vi "GOOP_AllVIs.vi"   [LabVIEW 2020]
uses:
  <resource>/Framework/Providers/Open_GDS/SubVIs/GOOP_HelpButton.ctl
  <resource>/Framework/Providers/Open_GDS/SubVIs/GOOP_MethodArgumentConnectionType.ctl
  <resource>/Framework/Providers/Open_GDS/ClassProviders/Common/CommonVIs/CommonVIs_AttributeDataType.ctl
  <resource>/Framework/Providers/Open_GDS/SubVIs/GOOP_MethodArgumentType.ctl
  <resource>/Framework/Providers/Open_GDS/SubVIs/GOOP_ProductType.ctl
  <resource>/Framework/Providers/Open_GDS/SubVIs/GOOP_ToolVersion.vi
  <resource>/Framework/Providers/Open_GDS/SubVIs/GOOP_UMLEditor_CallMainAction.ctl
  <resource>/Framework/Providers/Open_GDS/SubVIs/GOOP_WirePattern.ctl
  <resource>/Framework/Providers/Open_GDS/SubVIs/GOOP_WireConfigurationType.ctl
  <resource>/Framework/Providers/Open_GDS/ClassProviders/Provider_EndevoGOOP300/ClassWriterGOOP300_class/ClassWriterGOOP300.lvclass
  <resource>/Framework/Providers/Open_GDS/SubVIs/GOOP_ClassProviderClassType.ctl
  <resource>/Framework/Providers/Open_GDS/SubVIs/GOOP_ClassSettingsMemory_Action.ctl
  <resource>/Framework/Providers/Open_GDS/ClassProviders/Provider_LvNativeClass/ClassWriterNative_class/ClassWriterNative.lvclass
  <resource>/Framework/Providers/Open_GDS/SubVIs/GOOP_ErrorCodes.ctl
types:
  T1 = typedef "GOOP_ErrorCodes.ctl" = enum16{"LicenseFileMissing", "LicenseFileNotCorrect", "NoProductAccessGranted", "AgreementNoAccepted", "NoValidProviderFound", "LicenseExpired", "LanguageUndefined", "LanguageFileMissing", "LanguageFileChecksumError", "DublicateLanguageTranslation", "LanguageStringIDNotFound", "CommunityLimitReached", "ClassFileLocked", "ClassFileReadOnly", "ProjectNotValid"}
  T2 = typedef "GOOP_ClassSettingsMemory_Action.ctl" = enum16{"Read", "Write", "Read (ClassItemIconOnly)"}
  T3 = typedef "GOOP_ClassProviderClassType.ctl" = enum16{"ClassWriter", "ClassReader"}
  T4 = typedef "GOOP_WirePattern.ctl" = enum16{"Solid", "Large dash", "Small dash"}
  T5 = typedef "GOOP_WireConfigurationType.ctl" = cluster{"Edge thickness":i32, "Edge color":u32, "Center thickness":i32, "Center pattern":T4, "CenterColor1":u32, "CenterColor2":u32, "Tunnels and terminals colors":u32}
  T6 = typedef "GOOP_UMLEditor_CallMainAction.ctl" = enum16{"OpenUmlEditor", "ReverseEngineering:WholeProject", "ReverseEngineering:OneClass", "ReverseEngineering:OneVI", "ShowInStateDiagram:OneVI", "OpenUMLFile"}
  T7 = typedef "GOOP_ProductType.ctl" = enum16{"InvalidType", "Community Edition", "Professional Edition", "UML Community Edition", "UML Architect Edition"}
  T8 = typedef "GOOP_MethodArgumentType.ctl" = cluster{"Name":string, "DataType":T9, "ArrayDimensions":u8, "ConnectionType":T10, "DataTypeReference":path}
  T9 = typedef "CommonVIs_AttributeDataType.ctl" = enum16{"UINT8", "INT8", "UINT16", "INT16", "UINT32", "INT32", "UINT64", "INT64", "SGL", "DBL", "EXT", "CSG", "CDB", "CXT", "TimeStamp", "STRING", "PATH", "BOOL", "ENUM", "RefNum", "VIRefNum", "LabVIEW Class", "Cluster", "Variant", "TypeDef", "Waveform", "LabVIEW Object", "Other", "void", "Set", "Map"}
  T10 = typedef "GOOP_MethodArgumentConnectionType.ctl" = enum16{"Required", "Recommended", "Optional", "Dynamic Dispatch"}
  T11 = typedef "GOOP_HelpButton.ctl" = bool
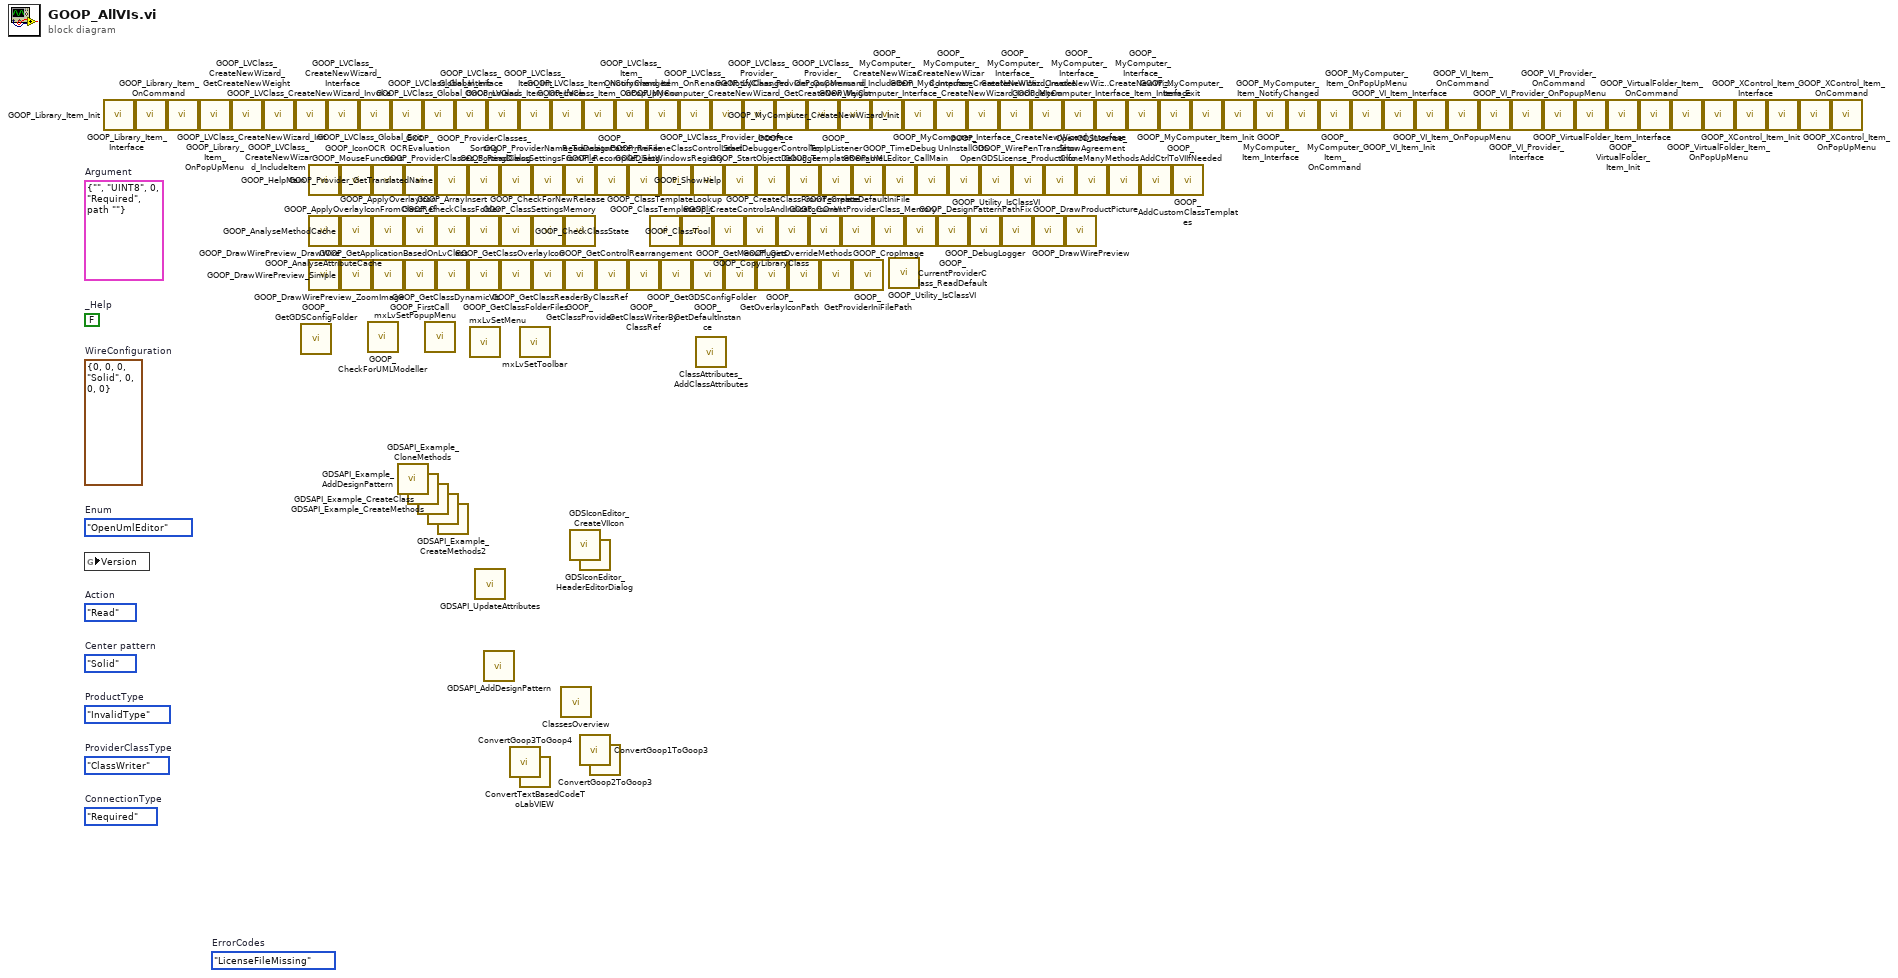
[diagram p0: block diagram]
diagram:
  (unwired) GOOP_ErrorCodes."LicenseFileMissing"  # ErrorCodes
  (unwired) GOOP_ClassSettingsMemory_Action."Read"  # Action
  (unwired) GOOP_ClassProviderClassType."ClassWriter"  # ProviderClassType
  (unwired) GOOP_WirePattern."Solid"  # Center pattern
  (unwired) T5 {"Edge thickness"=0, "Edge color"=0, "Center thickness"=0, "Center pattern"=enum."Solid", "CenterColor1"=0, "CenterColor2"=0, "Tunnels and terminals colors"=0}  # WireConfiguration
  (unwired) GOOP_UMLEditor_CallMainAction."OpenUmlEditor"  # Enum
  (unwired) GOOP_ProductType."InvalidType"  # ProductType
  (unwired) T8 {"Name"="", "DataType"=enum."UINT8", "ArrayDimensions"=0, "ConnectionType"=enum."Required", "DataTypeReference"=path ""}  # Argument
  (unwired) GOOP_MethodArgumentConnectionType."Required"  # ConnectionType
  (unwired) T11 FALSE  # _Help
  n1 = global read "GOOP_ToolVersion.vi" "Version"() -> ()  [unwired: 1 in]
  n2 = call <resource>:"GOOP_Library_Item_Init.vi"() -> ()  [unwired: 12 in]
  n3 = call <resource>:"GOOP_Library_Item_Interface.vi"() -> ()  [unwired: 11 in, 1 out]
  n4 = call <resource>:"GOOP_Library_Item_OnCommand.vi"() -> ()  [unwired: 12 in]
  n5 = call <resource>:"GOOP_Library_Item_OnPopUpMenu.vi"() -> ()  [unwired: 12 in]
  n6 = call <resource>:"GOOP_LVClass_CreateNewWizard_GetCreateNewWeight.vi"() -> ()  [unwired: 11 in, 1 out]
  n7 = call <resource>:"GOOP_LVClass_CreateNewWizard_IncludeItem.vi"() -> ()  [unwired: 11 in, 1 out]
  n8 = call <resource>:"GOOP_LVClass_CreateNewWizard_Init.vi"() -> ()  [unwired: 9 in, 3 out]
  n9 = call <resource>:"GOOP_GetGDSConfigFolder.vi"() -> ()  [unwired: 1 out]
  n10 = call <resource>:"GOOP_HelpMain.vi"() -> ()  [unwired: 12 in]
  n11 = call <resource>:"GOOP_AnalyseAttributeCache.vi"() -> ()  [unwired: 9 in, 3 out]
  n12 = call <resource>:"GOOP_DrawWirePreview_DrawWire.vi"() -> ()  [unwired: 11 in, 1 out]
  n13 = call <resource>:"GOOP_LVClass_CreateNewWizard_Interface.vi"() -> ()  [unwired: 11 in, 1 out]
  n14 = call <resource>:"GOOP_IconOCR.vi"() -> ()  [unwired: 11 in, 1 out]
  n15 = call <resource>:"GOOP_AnalyseMethodCache.vi"() -> ()  [unwired: 9 in, 3 out]
  n16 = call <resource>:"GOOP_DrawWirePreview_Simple.vi"() -> ()  [unwired: 7 in, 5 out]
  n17 = call <resource>:"GOOP_LVClass_CreateNewWizard_Invoke.vi"() -> ()  [unwired: 11 in, 1 out]
  n18 = call <resource>:"GOOP_CheckForUMLModeller.vi"() -> ()  [unwired: 10 in, 2 out]
  n19 = call <resource>:"GOOP_MouseFunctions.vi"() -> ()  [unwired: 9 in, 3 out]
  n20 = call <resource>:"GOOP_ApplyOverlayIcon.vi"() -> ()  [unwired: 11 in, 1 out]
  n21 = call <resource>:"GOOP_DrawWirePreview_ZoomImage.vi"() -> ()  [unwired: 2 in, 1 out]
  n22 = call <resource>:"GOOP_LVClass_Global_Exit.vi"() -> ()  [unwired: 12 in]
  n23 = call <resource>:"GDSAPI_Example_AddDesignPattern.vi"() -> ()  [unwired: 12 in]
  n24 = call <resource>:"GOOP_OCREvaluation.vi"() -> ()  [unwired: 11 in, 1 out]
  n25 = call <resource>:"GOOP_ApplyOverlayIconFromClassRef.vi"() -> ()  [unwired: 11 in, 1 out]
  n26 = call <resource>:"GOOP_FirstCall.vi"() -> ()  [unwired: 11 in, 1 out]
  n27 = call <resource>:"GDSAPI_Example_CloneMethods.vi"() -> ()  [unwired: 12 in]
  n28 = call <resource>:"GDSAPI_Example_CreateClass.vi"() -> ()  [unwired: 12 in]
  n29 = call <resource>:"GOOP_LVClass_Global_Init.vi"() -> ()  [unwired: 12 in]
  n30 = call <resource>:"mxLvSetPopupMenu.vi"() -> ()  [unwired: 10 in, 2 out]
  n31 = call <resource>:"GDSAPI_Example_CreateMethods.vi"() -> ()  [unwired: 12 in]
  n32 = call <resource>:"GOOP_Provider_GetTranslatedName.vi"() -> ()  [unwired: 11 in, 1 out]
  n33 = call <resource>:"GOOP_ArrayInsert.vi"() -> ()  [unwired: 19 in, 1 out]
  n34 = call <resource>:"GOOP_GetApplicationBasedOnLvClass.vi"() -> ()  [unwired: 10 in, 2 out]
  n35 = call <resource>:"GDSAPI_Example_CreateMethods2.vi"() -> ()  [unwired: 12 in]
  n36 = call <resource>:"GOOP_LVClass_Global_Interface.vi"() -> ()  [unwired: 11 in, 1 out]
  n37 = call <resource>:"GOOP_ProviderClasses_Sorting.vi"() -> ()  [unwired: 9 in, 3 out]
  n38 = call <resource>:"GOOP_CheckClassFolder.vi"() -> ()  [unwired: 7 in, 5 out]
  n39 = call <resource>:"GOOP_GetClassDynamicVIs.vi"() -> ()  [unwired: 12 in, 8 out]
  n40 = call <resource>:"mxLvSetMenu.vi"() -> ()  [unwired: 10 in, 2 out]
  n41 = call <resource>:"GDSAPI_UpdateAttributes.vi"() -> ()  [unwired: 11 in, 1 out]
  n42 = call <resource>:"GDSAPI_AddDesignPattern.vi"() -> ()  [unwired: 11 in, 1 out]
  n43 = call <resource>:"GOOP_LVClass_Global_OnCommand.vi"() -> ()  [unwired: 12 in]
  n44 = call <resource>:"GOOP_ProviderClasses_SortingDialog.vi"() -> ()  [unwired: 9 in, 3 out]
  n45 = call <resource>:"GOOP_CheckClassState.vi"() -> ()  [unwired: 11 in, 1 out]
  n46 = call <resource>:"GOOP_GetClassFolderFiles.vi"() -> ()  [unwired: 11 in, 1 out]
  n47 = call <resource>:"ConvertGoop3ToGoop4.vi"() -> ()  [unwired: 11 in, 1 out]
  n48 = call <resource>:"GOOP_LVClass_Item_Init.vi"() -> ()  [unwired: 12 in]
  n49 = call <resource>:"mxLvSetToolbar.vi"() -> ()  [unwired: 10 in, 2 out]
  n50 = call <resource>:"ConvertTextBasedCodeToLabVIEW.vi"() -> ()  [unwired: 12 in]
  n51 = call <resource>:"GOOP_ProviderName_Translator.vi"() -> ()  [unwired: 11 in, 1 out]
  n52 = call <resource>:"GOOP_CheckForNewRelease.vi"() -> ()  [unwired: 12 in]
  n53 = call <resource>:"GOOP_GetClassOverlayIcon.vi"() -> ()  [unwired: 9 in, 3 out]
  n54 = call <resource>:"GOOP_LVClass_Item_Interface.vi"() -> ()  [unwired: 11 in, 1 out]
  n55 = call <resource>:"ClassesOverview.vi"() -> ()  [unwired: 11 in, 1 out]
  n56 = call <resource>:"GOOP_ReadClassSettingsFromFile.vi"() -> ()  [unwired: 9 in, 3 out]
  n57 = call <resource>:"GOOP_ClassSettingsMemory.vi"() -> ()  [unwired: 14 in, 6 out]
  n58 = call <resource>:"GOOP_GetClassProvider.vi"() -> ()  [unwired: 17 in, 3 out]
  n59 = call <resource>:"GDSIconEditor_CreateVIIcon.vi"() -> ()  [unwired: 11 in, 1 out]
  n60 = call <resource>:"GDSIconEditor_HeaderEditorDialog.vi"() -> ()  [unwired: 15 in, 5 out]
  n61 = call <resource>:"ConvertGoop1ToGoop3.vi"() -> ()  [unwired: 11 in, 1 out]
  n62 = call <resource>:"GOOP_LVClass_Item_NotifyChanged.vi"() -> ()  [unwired: 12 in]
  n63 = call <resource>:"ConvertGoop2ToGoop3.vi"() -> ()  [unwired: 11 in, 1 out]
  n64 = call <resource>:"GOOP_ReadDesignPatternIniFile.vi"() -> ()  [unwired: 10 in, 2 out]
  n65 = call <resource>:"GOOP_GetClassReaderByClassRef.vi"() -> ()  [unwired: 18 in, 2 out]
  n66 = call <resource>:"GOOP_LVClass_Item_OnCommand.vi"() -> ()  [unwired: 12 in]
  n67 = call <resource>:"GOOP_RecompileDialog.vi"() -> ()  [unwired: 19 in, 1 out]
  n68 = call <resource>:"GOOP_GetClassWriterByClassRef.vi"() -> ()  [unwired: 18 in, 2 out]
  n69 = call <resource>:"GOOP_LVClass_Item_OnPopUpMenu.vi"() -> ()  [unwired: 12 in]
  n70 = call <resource>:"GOOP_ClassTemplateLookup.vi"() -> ()  [unwired: 11 in, 1 out]
  n71 = call <resource>:"GOOP_RenameClassControlLabel.vi"() -> ()  [unwired: 10 in, 2 out]
  n72 = call <resource>:"GOOP_GetControlRearrangement.vi"() -> ()  [unwired: 13 in, 7 out]
  n73 = call <resource>:"GOOP_LVClass_Item_OnRename.vi"() -> ()  [unwired: 12 in]
  n74 = call <resource>:"GOOP_ClassTemplateSplit.vi"() -> ()  [unwired: 14 in, 2 out]
  n75 = call <resource>:"GOOP_SetWindowsRegistry.vi"() -> ()  [unwired: 11 in, 1 out]
  n76 = call <resource>:"GOOP_GetDefaultInstance.vi"() -> ()  [unwired: 9 in, 3 out]
  n77 = call <resource>:"ClassAttributes_AddClassAttributes.vi"() -> ()  [unwired: 8 in, 4 out]
  n78 = call <resource>:"GOOP_LVClass_Provider_Interface.vi"() -> ()  [unwired: 11 in, 1 out]
  n79 = call <resource>:"GOOP_ClassTool.vi"() -> ()  [unwired: 19 in, 1 out]
  n80 = call <resource>:"GOOP_ShowHelp.vi"() -> ()  [unwired: 1 in]
  n81 = call <resource>:"GOOP_GetGDSConfigFolder.vi"() -> ()  [unwired: 1 out]
  n82 = call <resource>:"GOOP_LVClass_Provider_NotifyChanged.vi"() -> ()  [unwired: 12 in]
  n83 = call <resource>:"GOOP_CopyLibraryClass.vi"() -> ()  [unwired: 9 in, 3 out]
  n84 = call <resource>:"GOOP_StartDebuggerController.vi"() -> ()  [unwired: 19 in, 1 out]
  n85 = call <resource>:"GOOP_GetMenuPlugins.vi"() -> ()  [unwired: 10 in, 2 out]
  n86 = call <resource>:"GOOP_LVClass_Provider_OnCommand.vi"() -> ()  [unwired: 12 in]
  n87 = call <resource>:"GOOP_CreateClassFromTemplate.vi"() -> ()  [unwired: 12 in, 8 out]
  n88 = call <resource>:"GOOP_StartObjectDebugger.vi"() -> ()  [unwired: 19 in, 1 out]
  n89 = call <resource>:"GOOP_GetOverlayIconPath.vi"() -> ()  [unwired: 11 in, 1 out]
  n90 = call <resource>:"GOOP_LVClass_Provider_OnPopupMenu.vi"() -> ()  [unwired: 12 in]
  n91 = call <resource>:"GOOP_CreateControlsAndIndicatorsOnVI.vi"() -> ()  [unwired: 11 in, 1 out]
  n92 = call <resource>:"GOOP_TcpIpListener.vi"() -> ()  [unwired: 12 in]
  n93 = call <resource>:"GOOP_GetOverrideMethods.vi"() -> ()  [unwired: 14 in, 6 out]
  n94 = call <resource>:"GOOP_MyComputer_CreateNewWizard_GetCreateNewWeight.vi"() -> ()  [unwired: 11 in, 1 out]
  n95 = call <resource>:"GOOP_CreateDefaultIniFile.vi"() -> ()  [unwired: 10 in, 2 out]
  n96 = call <resource>:"GOOP_TemplateRename.vi"() -> ()  [unwired: 11 in, 1 out]
  n97 = call <resource>:"GOOP_GetProviderIniFilePath.vi"() -> ()  [unwired: 10 in, 2 out]
  n98 = call <resource>:"GOOP_MyComputer_CreateNewWizard_IncludeItem.vi"() -> ()  [unwired: 11 in, 1 out]
  n99 = call <resource>:"GOOP_CropImage.vi"() -> ()  [unwired: 6 in, 2 out]
  n100 = call <resource>:"GOOP_TimeDebug.vi"() -> ()  [unwired: 12 in]
  n101 = call <resource>:"GOOP_Utility_IsClassVI.vi"() -> ()  [unwired: 6 in, 6 out]
  n102 = call <resource>:"GOOP_MyComputer_CreateNewWizard_Init.vi"() -> ()  [unwired: 9 in, 3 out]
  n103 = call <resource>:"GOOP_CurrentProviderClass_Memory.vi"() -> ()  [unwired: 13 in, 7 out]
  n104 = call <resource>:"GOOP_UMLEditor_CallMain.vi"() -> ()  [unwired: 19 in, 1 out]
  n105 = call <resource>:"GOOP_MyComputer_CreateNewWizard_Interface.vi"() -> ()  [unwired: 11 in, 1 out]
  n106 = call <resource>:"GOOP_CurrentProviderClass_ReadDefault.vi"() -> ()  [unwired: 11 in, 5 out]
  n107 = call <resource>:"GOOP_UnInstallGDS.vi"() -> ()  [unwired: 19 in, 1 out]
  n108 = call <resource>:"GOOP_MyComputer_CreateNewWizard_Invoke.vi"() -> ()  [unwired: 11 in, 1 out]
  n109 = call <resource>:"GOOP_DebugLogger.vi"() -> ()  [unwired: 9 in, 3 out]
  n110 = call <resource>:"GOOP_Utility_IsClassVI.vi"() -> ()  [unwired: 6 in, 6 out]
  n111 = call <resource>:"GOOP_MyComputer_Interface_CreateNewWizard_GetCreateNewWeight.vi"() -> ()  [unwired: 11 in, 1 out]
  n112 = call <resource>:"GOOP_DesignPatternPathFix.vi"() -> ()  [unwired: 7 in, 5 out]
  n113 = call <resource>:"GOOP_WirePenTranslator.vi"() -> ()  [unwired: 18 in, 2 out]
  n114 = call <resource>:"GOOP_MyComputer_Interface_CreateNewWizard_IncludeItem.vi"() -> ()  [unwired: 11 in, 1 out]
  n115 = call <resource>:"GOOP_DrawProductPicture.vi"() -> ()  [unwired: 11 in, 1 out]
  n116 = call <resource>:"OpenGDSLicense_ProductInfo.vi"() -> ()  [unwired: 19 in, 1 out]
  n117 = call <resource>:"GOOP_MyComputer_Interface_CreateNewWizard_Init.vi"() -> ()  [unwired: 9 in, 3 out]
  n118 = call <resource>:"GOOP_DrawWirePreview.vi"() -> ()  [unwired: 18 in, 2 out]
  n119 = call <resource>:"OpenGDSLicense_ShowAgreement.vi"() -> ()  [unwired: 18 in, 2 out]
  n120 = call <resource>:"GOOP_MyComputer_Interface_CreateNewWizard_Interface.vi"() -> ()  [unwired: 11 in, 1 out]
  n121 = call <resource>:"CloneManyMethods.vi"() -> ()  [unwired: 18 in, 2 out]
  n122 = call <resource>:"GOOP_MyComputer_Interface_CreateNewWizard_Invoke.vi"() -> ()  [unwired: 11 in, 1 out]
  n123 = call <resource>:"GOOP_AddCtrlToVIIfNeeded.vi"() -> ()  [unwired: 9 in, 3 out]
  n124 = call <resource>:"GOOP_MyComputer_Interface_Item_Interface.vi"() -> ()  [unwired: 11 in, 1 out]
  n125 = call <resource>:"GOOP_AddCustomClassTemplates.vi"() -> ()  [unwired: 2 in, 1 out]
  n126 = call <resource>:"GOOP_MyComputer_Item_Exit.vi"() -> ()  [unwired: 12 in]
  n127 = call <resource>:"GOOP_MyComputer_Item_Init.vi"() -> ()  [unwired: 12 in]
  n128 = call <resource>:"GOOP_MyComputer_Item_Interface.vi"() -> ()  [unwired: 11 in, 1 out]
  n129 = call <resource>:"GOOP_MyComputer_Item_NotifyChanged.vi"() -> ()  [unwired: 12 in]
  n130 = call <resource>:"GOOP_MyComputer_Item_OnCommand.vi"() -> ()  [unwired: 12 in]
  n131 = call <resource>:"GOOP_MyComputer_Item_OnPopUpMenu.vi"() -> ()  [unwired: 12 in]
  n132 = call <resource>:"GOOP_VI_Item_Init.vi"() -> ()  [unwired: 12 in]
  n133 = call <resource>:"GOOP_VI_Item_Interface.vi"() -> ()  [unwired: 11 in, 1 out]
  n134 = call <resource>:"GOOP_VI_Item_OnCommand.vi"() -> ()  [unwired: 12 in]
  n135 = call <resource>:"GOOP_VI_Item_OnPopupMenu.vi"() -> ()  [unwired: 12 in]
  n136 = call <resource>:"GOOP_VI_Provider_Interface.vi"() -> ()  [unwired: 11 in, 1 out]
  n137 = call <resource>:"GOOP_VI_Provider_OnCommand.vi"() -> ()  [unwired: 12 in]
  n138 = call <resource>:"GOOP_VI_Provider_OnPopupMenu.vi"() -> ()  [unwired: 12 in]
  n139 = call <resource>:"GOOP_VirtualFolder_Item_Init.vi"() -> ()  [unwired: 12 in]
  n140 = call <resource>:"GOOP_VirtualFolder_Item_Interface.vi"() -> ()  [unwired: 11 in, 1 out]
  n141 = call <resource>:"GOOP_VirtualFolder_Item_OnCommand.vi"() -> ()  [unwired: 12 in]
  n142 = call <resource>:"GOOP_VirtualFolder_Item_OnPopUpMenu.vi"() -> ()  [unwired: 12 in]
  n143 = call <resource>:"GOOP_XControl_Item_Init.vi"() -> ()  [unwired: 12 in]
  n144 = call <resource>:"GOOP_XControl_Item_Interface.vi"() -> ()  [unwired: 11 in, 1 out]
  n145 = call <resource>:"GOOP_XControl_Item_OnCommand.vi"() -> ()  [unwired: 12 in]
  n146 = call <resource>:"GOOP_XControl_Item_OnPopUpMenu.vi"() -> ()  [unwired: 12 in]
